vi "CMD_DBLOGIN.vi"(6 "Gantry in":refnum<class "Gantry.lvclass">, 8 "error in (no error)":errorcluster, 10 "Arguments":string[](array[string]), 11 "gScript Interpreter in":refnum<class "gScript Interpreter.lvclass">) -> (0 "error out":errorcluster, 3 "gScript Interpreter out":refnum<class "gScript Interpreter.lvclass">, 4 "Gantry out":refnum<class "Gantry.lvclass">)   [LabVIEW 2017, in "gScript Interpreter.lvclass"]
uses:
  gScript Interpreter.lvclass
  Shared Components/Gantry Class/Gantry.lvclass
  <vilib>/Utility/config.llb/Read Key (String).vi
  <vilib>/Utility/config.llb/Read Key (I32).vi
  <vilib>/Utility/config.llb/Write Key (String).vi
  <vilib>/Utility/config.llb/Write Key (I32).vi
  Shared Components/FlexWorktable/FlexWorktable.lvclass
  Shared Components/External/Database/Database.lvlib
  <vilib>/Utility/config.llb/NI_LVConfig.lvlib
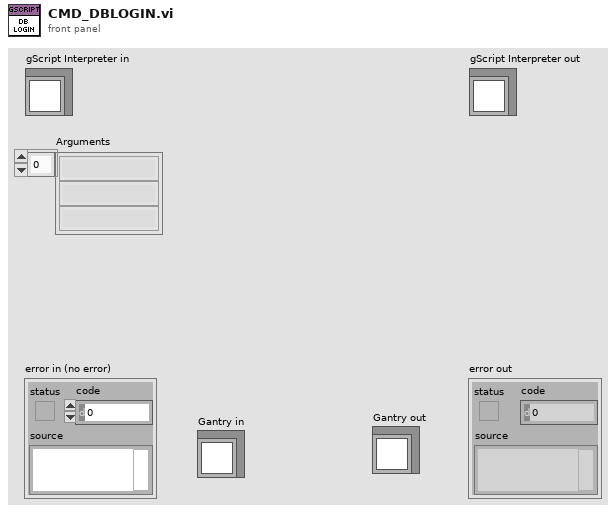
[diagram p1: front panel]
types:
  T1 = typedef "NI_LVConfig.lvlib/Config Data RefNum.ctl" = refnum<k1>
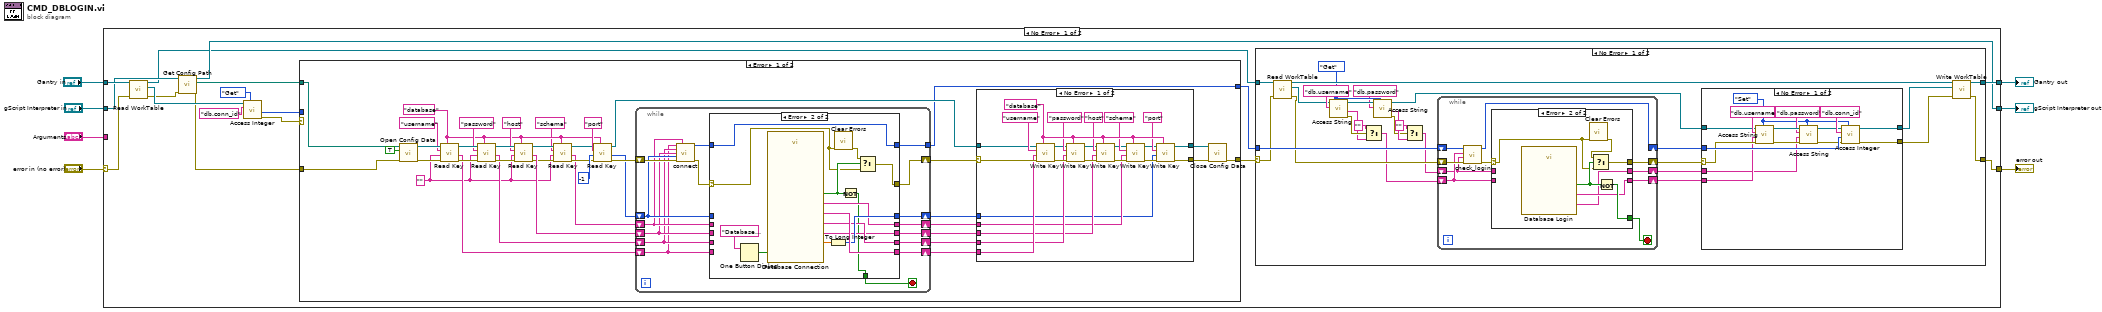
[diagram p0: block diagram]
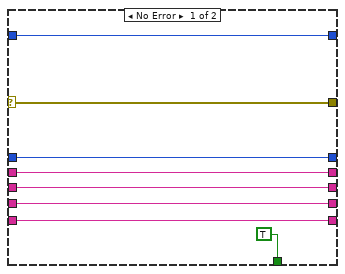
[diagram p3: hidden frame]
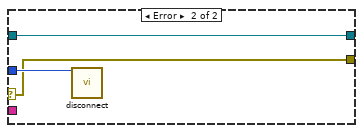
[diagram p5: hidden frame]
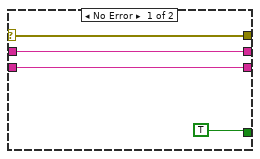
[diagram p6: hidden frame]
diagram:
  n1 = case shown="No Error" "error in (no error)" {
    selector: "error in (no error)" -> [w19 w198]
    tunnel: [w23 w198] -> w6
    tunnel: [w12 w197] -> w4
    tunnel: "gScript Interpreter in" -> [w13 w197]
    tunnel: "Arguments" -> [_ _]
    tunnel: "Gantry in" -> [w20 w196]
    tunnel: [w24 w196] -> w1
    frame No Error {
      n2 = call-dynamic "Read WorkTable.vi"("error in"=w19, "Gantry Class in"=w20) -> ("error out"=w11:errorcluster, "Worktable"=w18:refnum<class "FlexWorktable.lvclass">, "Gantry Class out"=w8:refnum<class "Gantry.lvclass">)  [unwired: 7 in]
      n3 = call "Get Config Path.vi"("error in (no error)"=w11, "gScript Interpreter in"=w13) -> ("error out"=w10:errorcluster, "INI Config Path"=w9:path, "gScript Interpreter out"=w12:refnum<class "gScript Interpreter.lvclass">)  [unwired: 7 in]
      n4 = call-dynamic "Access Integer.vi"("Get/Set"=enum16{"Get", "Set"}."Get", "Key"="db.conn_id", "FlexWorktable in"=w18) -> ("error out"=w14:errorcluster, "Value out"=w15:i32)  [unwired: 6 in, 1 out]
      n5 = case shown="Error" w14 {
        tunnel: w10 -> [w58 w126]
        tunnel: [w27 w126] -> w22
        tunnel: [w26 w127] -> w21
        tunnel: w15 -> [_ w127]
        tunnel: w9 -> [w25 _]
        frame Error {
          w38 = "" ("default value")
          w40 = "database" ("section")
          n6 = call <vilib>:"Open Config Data.vi"("error in (no error)"=w58, "create file if necessary (T)"=TRUE, "configuration file path"=w25) -> ("error out"=w61:errorcluster, "refnum"=w60:T1)  [unwired: 6 in, 1 out]
          n7 = call-poly <vilib>:"Read Key.vi"("section"=w40, "error in (no error)"=w61, "default value"=w38, "key"="username", "refnum"=w60) -> ("error out"=w57:errorcluster, "value"=w49:string, "refnum out"=w54:T1)  [unwired: 3 in, 1 out]
          n8 = call-poly <vilib>:"Read Key.vi"("section"=w40, "error in (no error)"=w57, "default value"=w38, "key"="password", "refnum"=w54) -> ("error out"=w56:errorcluster, "value"=w48:string, "refnum out"=w55:T1)  [unwired: 3 in, 1 out]
          n9 = call-poly <vilib>:"Read Key.vi"("section"=w40, "error in (no error)"=w56, "default value"=w38, "key"="host", "refnum"=w55) -> ("error out"=w42:errorcluster, "value"=w47:string, "refnum out"=w44:T1)  [unwired: 3 in, 1 out]
          n10 = call-poly <vilib>:"Read Key.vi"("section"=w40, "error in (no error)"=w42, "default value"=w38, "key"="schema", "refnum"=w44) -> ("error out"=w41:errorcluster, "value"=w37:string, "refnum out"=w43:T1)  [unwired: 3 in, 1 out]
          n11 = call-poly <vilib>:"Read Key.vi"("section"=w40, "error in (no error)"=w41, "default value"=-1, "key"="port", "refnum"=w43) -> ("error out"=w50:errorcluster, "value"=w46:i32, "refnum out"=w35:T1)  [unwired: 3 in, 1 out]
          n12 = while {
            shift-right: [w97] -> w34
            shift-left: w46 -> [w96]
            shift-right: [w92] -> w32
            shift-left: w47 -> [w93]
            shift-right: [w90] -> w31
            shift-left: w48 -> [w91]
            shift-right: [w98] -> w30
            shift-left: w49 -> [w89]
            shift-right: [w94] -> w33
            shift-left: w37 -> [w95]
            tunnel: [w100] -> w26
            shift-right: [w88] -> w36
            shift-left: w50 -> [w103]
            stop <- w99 stop-if-true
            n13 = call "connect.vi"("username"=w89, "schema"=w95, "password"=w91, "host"=w93, "port"=w96, "error in (no error)"=w103) -> ("DB Session ID"=w101:i32, "error out"=w102:errorcluster)  [unwired: 8 in]
            n14 = case shown="Error" w102 {
              selector: w102 -> [w104 w113]
              tunnel: w101 -> [w111 w119]
              tunnel: [w111 w119] -> w100
              tunnel: [TRUE w116] -> w99
              tunnel: [w105 w124] -> w98
              tunnel: [w109 w123] -> w97
              tunnel: w96 -> [w109 _]
              tunnel: w95 -> [w108 _]
              tunnel: [w108 w120] -> w94
              tunnel: w93 -> [w107 _]
              tunnel: [w107 w121] -> w92
              tunnel: w91 -> [w106 _]
              tunnel: [w106 w122] -> w90
              tunnel: w89 -> [w105 _]
              tunnel: [w104 w112] -> w88
              frame No Error {
              }
              frame Error {
                n15 = One Button Dialog(message="Database Connection Failed" ("host")) -> (true=w117:bool)  [unwired: 1 in]
                n16 = call "Database Connection"("Enable"=w117) -> ("port"=w125:dbl, "schema"=w120:string, "host"=w121:string, "password"=w122:string, "username"=w124:string, "OK"=w114:bool)  [unwired: 12 in, 1 out]
                n17 = To Long Integer(number=w125) -> (32bit integer=w123:i32)
                n18 = call <vilib>:"Clear Errors.vi"("error in (no error)"=w113) -> ("error out"=w115:errorcluster)  [unwired: 5 in, 1 out]
                n19 = Not(x=w114) -> (.not. x?=w116:bool)
                n20 = Select(t=w115, s=w114, f=w113) -> (s? t:f=w112:errorcluster)
              }
            }
          }
          n21 = case shown="No Error" w36 {
            selector: w36 -> [w85 w86]
            tunnel: w35 -> [w72 w87]
            tunnel: [w79 w86] -> w28
            tunnel: w34 -> [w68 _]
            tunnel: w33 -> [w69 _]
            tunnel: w32 -> [w70 _]
            tunnel: w31 -> [w71 _]
            tunnel: w30 -> [w73 _]
            tunnel: [w63 w87] -> w29
            frame No Error {
              w84 = "database" ("section")
              n22 = call-poly <vilib>:"Write Key.vi"("section"=w84, "error in (no error)"=w85, "value"=w73, "key"="username", "refnum"=w72) -> ("error out"=w83:errorcluster, "refnum out"=w67:T1)  [unwired: 4 in, 1 out]
              n23 = call-poly <vilib>:"Write Key.vi"("section"=w84, "error in (no error)"=w83, "value"=w71, "key"="password", "refnum"=w67) -> ("error out"=w82:errorcluster, "refnum out"=w66:T1)  [unwired: 4 in, 1 out]
              n24 = call-poly <vilib>:"Write Key.vi"("section"=w84, "error in (no error)"=w82, "value"=w70, "key"="host", "refnum"=w66) -> ("error out"=w81:errorcluster, "refnum out"=w65:T1)  [unwired: 4 in, 1 out]
              n25 = call-poly <vilib>:"Write Key.vi"("section"=w84, "error in (no error)"=w81, "value"=w69, "key"="schema", "refnum"=w65) -> ("error out"=w80:errorcluster, "refnum out"=w64:T1)  [unwired: 4 in, 1 out]
              n26 = call-poly <vilib>:"Write Key.vi"("section"=w84, "error in (no error)"=w80, "value"=w68, "key"="port", "refnum"=w64) -> ("error out"=w79:errorcluster, "refnum out"=w63:T1)  [unwired: 4 in, 1 out]
            }
            frame Error {
            }
          }
          n27 = call <vilib>:"Close Config Data.vi"("error in (no error)"=w28, "refnum"=w29) -> ("error out"=w27:errorcluster)  [unwired: 8 in, 1 out]
        }
        frame No Error {
        }
      }
      n28 = case shown="No Error" w22 {
        selector: w22 -> [w149 w195]
        tunnel: w8 -> [w154 w194]
        tunnel: [w152 w194] -> w24
        tunnel: [w151 w195] -> w23
        tunnel: w21 -> [w150 _]
        frame No Error {
          w145 = enum16{"Get", "Set"}."Get" ("Get/Set")
          n29 = call-dynamic "Read WorkTable.vi"("error in"=w149, "Gantry Class in"=w154) -> ("error out"=w138:errorcluster, "Worktable"=w147:refnum<class "FlexWorktable.lvclass">, "Gantry Class out"=w153:refnum<class "Gantry.lvclass">)  [unwired: 7 in]
          n30 = call-dynamic "Access String.vi"("Get/Set"=w145, "Key"="db.username", "FlexWorktable in"=w147) -> ("error out"=w144:errorcluster, "Value out"=w143:string, "FlexWorktable out"=w146:refnum<class "FlexWorktable.lvclass">)  [unwired: 6 in]
          n31 = Select(t="", s=w144, f=w143) -> (s? t:f=w136:string)
          n32 = call-dynamic "Access String.vi"("Get/Set"=w145, "Key"="db.password", "FlexWorktable in"=w146) -> ("error out"=w139:errorcluster, "Value out"=w140:string, "FlexWorktable out"=w130:refnum<class "FlexWorktable.lvclass">)  [unwired: 6 in]
          n33 = Select(t="", s=w139, f=w140) -> (s? t:f=w135:string)
          n34 = while {
            shift-right: [w180] -> w133
            shift-left: w150 -> [w182]
            shift-right: [w174] -> w129
            shift-left: w135 -> [w175]
            shift-right: [w176] -> w128
            shift-left: w136 -> [w177]
            shift-right: [w178] -> w134
            shift-left: w138 -> [w181]
            stop <- w173 stop-if-true
            n35 = call "check_login.vi"("error in (no error)"=w181, "password"=w175, "username"=w177, "DB Session ID"=w182) -> ("error out"=w179:errorcluster, "DB Session ID out"=w180:i32)  [unwired: 6 in]
            n36 = case shown="Error" w179 {
              selector: w179 -> [w186 w190]
              tunnel: [w186 w189] -> w178
              tunnel: w177 -> [w185 _]
              tunnel: [w185 w188] -> w176
              tunnel: w175 -> [w184 _]
              tunnel: [w184 w187] -> w174
              tunnel: [TRUE w193] -> w173
              frame No Error {
              }
              frame Error {
                n37 = call "Database Login"() -> ("password"=w187:string, "username"=w188:string, "Connect"=w192:bool)  [unwired: 16 in, 1 out]
                n38 = call <vilib>:"Clear Errors.vi"("error in (no error)"=w190) -> ("error out"=w191:errorcluster)  [unwired: 5 in, 1 out]
                n39 = Select(t=w191, s=w192, f=w190) -> (s? t:f=w189:errorcluster)
                n40 = Not(x=w192) -> (.not. x?=w193:bool)
              }
            }
          }
          n41 = case shown="No Error" w134 {
            selector: w134 -> [w158 w170]
            tunnel: w133 -> [w167 w172]
            tunnel: [w169 w170] -> w132
            tunnel: [w168 w171] -> w131
            tunnel: w130 -> [w162 w171]
            tunnel: w129 -> [w155 _]
            tunnel: w128 -> [w156 _]
            frame No Error {
              w157 = enum16{"Get", "Set"}."Set" ("Get/Set")
              n42 = call-dynamic "Access String.vi"("Get/Set"=w157, "error in (no error)"=w158, "Value in"=w156, "Key"="db.username", "FlexWorktable in"=w162) -> ("error out"=w159:errorcluster, "FlexWorktable out"=w164:refnum<class "FlexWorktable.lvclass">)  [unwired: 4 in, 1 out]
              n43 = call-dynamic "Access String.vi"("Get/Set"=w157, "error in (no error)"=w159, "Value in"=w155, "Key"="db.password", "FlexWorktable in"=w164) -> ("error out"=w160:errorcluster, "FlexWorktable out"=w161:refnum<class "FlexWorktable.lvclass">)  [unwired: 4 in, 1 out]
              n44 = call-dynamic "Access Integer.vi"("Get/Set"=w157, "error in (no error)"=w160, "Value in"=w167, "Key"="db.conn_id", "FlexWorktable in"=w161) -> ("error out"=w169:errorcluster, "FlexWorktable out"=w168:refnum<class "FlexWorktable.lvclass">)  [unwired: 4 in, 1 out]
            }
            frame Error {
              n45 = call "disconnect.vi"("DB Session ID"=w172) -> ()  [unwired: 14 in, 1 out]
            }
          }
          n46 = call-dynamic "Write WorkTable.vi"("error in (no error)"=w132, "FlexWorktable"=w131, "Gantry Class in"=w153) -> ("error out"=w151:errorcluster, "Gantry Class out"=w152:refnum<class "Gantry.lvclass">)  [unwired: 7 in]
        }
        frame Error {
        }
      }
    }
    frame Error {
    }
  }
  "error out" <- w6
  "gScript Interpreter out" <- w4
  "Gantry out" <- w1
